vi "SmartAddObject.vi"(10 "New Object In":refnum<vi>, 11 "Scene Object In":refnum<vi>) -> (0 "error out":errorcluster, 3 "Scene Object Out":refnum<vi>)   [LabVIEW 2014]
uses:
  <vilib>/picture/3D Picture Control/Object/Add Object (no reference).vi
  <vilib>/picture/3D Picture Control/NI_3D Picture Control.lvlib
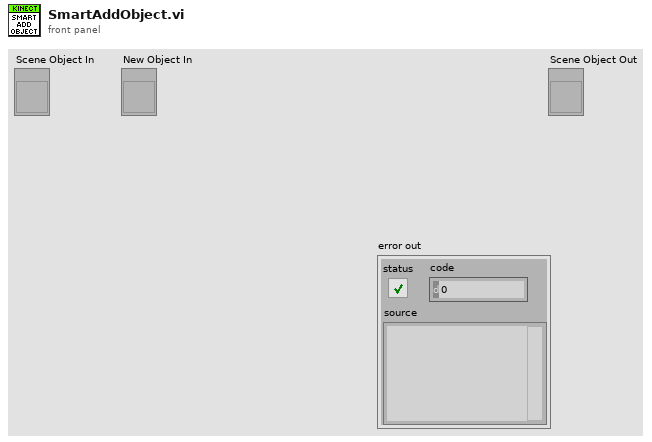
[diagram p1: front panel]
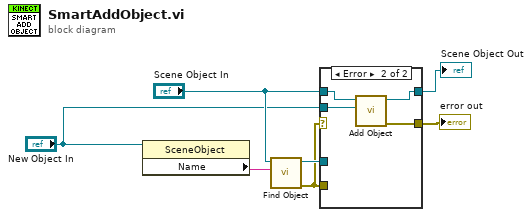
[diagram p0: block diagram]
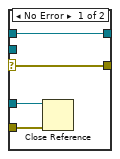
[diagram p2: hidden frame]
diagram:
  n1 = property class="SceneObject"(reference="New Object In") -> ("Name"=w7:string)  [unwired: 1 in, 2 out]
  n2 = call <vilib>:"Find Object.vi"("Object Name"=w7, "Scene Refnum"="Scene Object In") -> ("error out"=w1:errorcluster, "Object Refnum"=w2:refnum<vi>)  [unwired: 8 in]
  n3 = case shown="Error" w1 {
    selector: w1 -> [w10 _]
    tunnel: [w11 w13] -> w5
    tunnel: "Scene Object In" -> [w11 w15]
    tunnel: "New Object In" -> [_ w14]
    tunnel: [w10 w12] -> w4
    tunnel: w2 -> [w9 _]
    tunnel: w1 -> [w8 _]
    frame No Error {
      n4 = Close Reference(reference=w9, error in (no error)=w8) -> ()  [unwired: 1 out]
    }
    frame Error {
      n5 = call-poly <vilib>:"Add Object.vi"("New Object In"=w14, "Scene Object In"=w15) -> ("error out"=w12:errorcluster, "Scene Object Out"=w13:refnum<vi>)  [unwired: 8 in]
    }
  }
  "Scene Object Out" <- w5
  "error out" <- w4
